vi "_Logger.vi"(7 "Action":T1, 8 "Error In":errorcluster, 11 "Value In":variant) -> (0 "Error Out":errorcluster)   [LabVIEW 2015, in "Logger.lvlib"]
uses:
  Logger.lvlib
  _Logger Action.ctl
  Public/Controls/Message.ctl
  Public/Controls/Tag.ctl
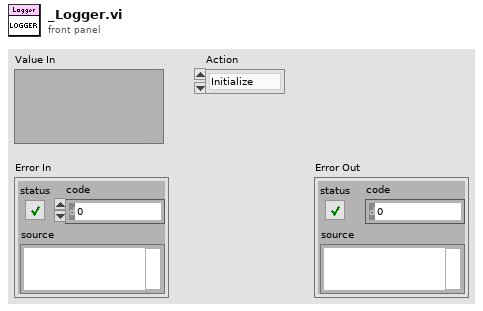
[diagram p1: front panel]
types:
  T1 = typedef "Logger.lvlib/_Logger Action.ctl" = enum16{"Initialize", "Register", "Log", "Unregister", "Set Level", "Shutdown"}
  T2 = typedef "Logger.lvlib/Message.ctl" = cluster{"Time Stamp":timestamp, "Tag":T3, "Source":string, "Text":string}
  T3 = typedef "Logger.lvlib/Tag.ctl" = enum16{"Fatal", "Error", "Warn", "Info", "Debug", "Trace"}
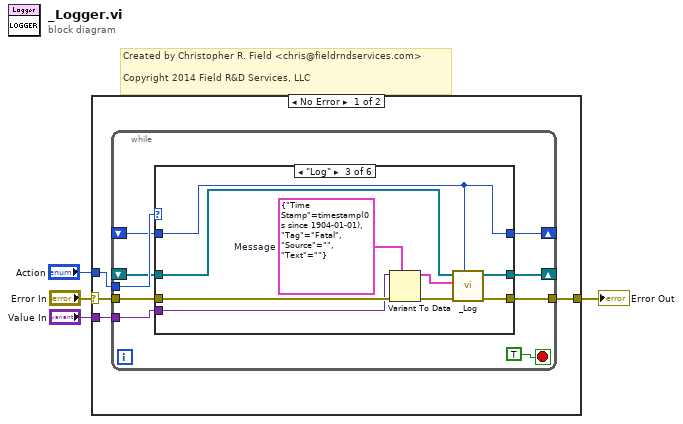
[diagram p0: block diagram]
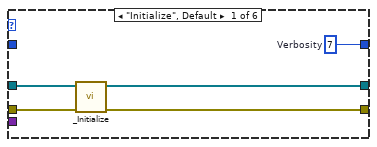
[diagram p2: hidden frame]
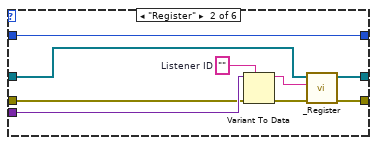
[diagram p3: hidden frame]
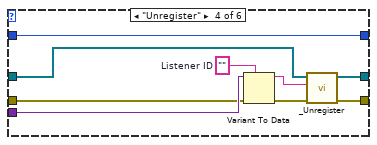
[diagram p4: hidden frame]
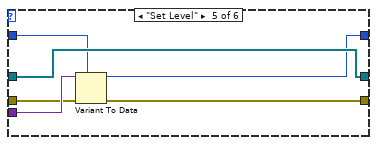
[diagram p5: hidden frame]
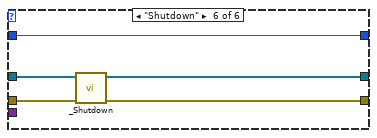
[diagram p6: hidden frame]
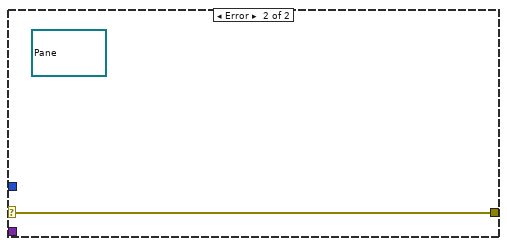
[diagram p7: hidden frame]
diagram:
  # "Created by Christopher R. Field <chris@fieldrndservices.com>\n\nCopyright 2014 Field R&D Services, LLC"
  n1 = case shown="No Error" "Error In" {
    selector: "Error In" -> [w7 w61]
    tunnel: [w6 w61] -> w3
    tunnel: "Action" -> [w8 _]
    tunnel: "Value In" -> [w5 _]
    frame No Error {
      n2 = while {
        tunnel: w8 -> [w16]
        tunnel: w7 -> [w15]
        tunnel: [w14] -> w6
        shift-right: [w13] -> _
        shift-left: _ -> [w12]
        tunnel: w5 -> [w11]
        shift-right: [w10] -> _
        shift-left: _ -> [w9]
        stop <- TRUE stop-if-true
        n3 = case shown="\"Log\"" w16 {
          tunnel: w15 -> [w20 w28 w39 w48 w54 w59]
          tunnel: [w19 w31 w40 w42 w52 w58] -> w14
          tunnel: [w22 w30 w34 w43 w53 w57] -> w13
          tunnel: w12 -> [w21 w25 w35 w44 w53 w60]
          tunnel: w11 -> [_ w29 w37 w49 w55 _]
          tunnel: [w18 w23 w32 w41 w50 w56] -> w10
          tunnel: w9 -> [_ w23 w32 w41 w51 w56]
          frame "Initialize", Default {
            w18 = u8 7  # Verbosity
            n4 = call "_Initialize.vi"("Error In"=w20, "Listeners In"=w21) -> ("Error Out"=w19:errorcluster, "Listeners Out"=w22:refnum<queue>[])  [unwired: 8 in]
          }
          frame "Register" {
            w26 = ""  # Listener ID
            n5 = Variant To Data(error in=w28, type=w26, Variant=w29) -> (data=w24:string, error out=w27:errorcluster)
            n6 = call "_Register.vi"("Error In"=w27, "Listener ID"=w24, "Listeners In"=w25) -> ("Error Out"=w31:errorcluster, "Listeners Out"=w30:refnum<queue>[])  [unwired: 7 in]
          }
          frame "Log" {
            w36 = T2 {"Time Stamp"=timestamp(0 s since 1904-01-01), "Tag"=enum."Fatal", "Source"="", "Text"=""}  # Message
            n7 = Variant To Data(error in=w39, type=w36, Variant=w37) -> (data=w33:T2, error out=w38:errorcluster)
            n8 = call "_Log.vi"("Level"=w32, "Error In"=w38, "Message"=w33, "Listeners In"=w35) -> ("Error Out"=w40:errorcluster, "Listeners Out"=w34:refnum<queue>[])  [unwired: 6 in]
          }
          frame "Unregister" {
            w47 = ""  # Listener ID
            n9 = Variant To Data(error in=w48, type=w47, Variant=w49) -> (data=w45:string, error out=w46:errorcluster)
            n10 = call "_Unregister.vi"("Error In"=w46, "Listener ID"=w45, "Listeners In"=w44) -> ("Error Out"=w42:errorcluster, "Listeners Out"=w43:refnum<queue>[])  [unwired: 7 in]
          }
          frame "Set Level" {
            n11 = Variant To Data(error in=w54, type=w51, Variant=w55) -> (data=w50:u8, error out=w52:errorcluster)
          }
          frame "Shutdown" {
            n12 = call "_Shutdown.vi"("Error In"=w59, "Listeners In"=w60) -> ("Error Out"=w58:errorcluster, "Listeners Out"=w57:refnum<queue>[])  [unwired: 8 in]
          }
        }
      }
    }
    frame Error {
      (unwired) refnum<user-event> refnum ("Log")
    }
  }
  "Error Out" <- w3
